vi "Open CANCoders.vi"(8 "error in":errorcluster, 11 "CANCoder Can IDs":T3={"LF ID"=12, "LB ID"=11, "RF ID"=10, "RB ID"=9}) -> (0 "error out":errorcluster, 3 "Swerve CANCoders":T1)   [LabVIEW 2020]
uses:
  Type Definitions/Hardware/4 Absolute Encoder Sets/(CANcoder) 4 Absolute Encoder Set.ctl
  <vilib>/Rock Robotics/WPI/ThirdParty/Phoenix-LabVIEW/CANCoder/Controls/CTRE_Phoenix_CANcoder_DeviceRef.ctl
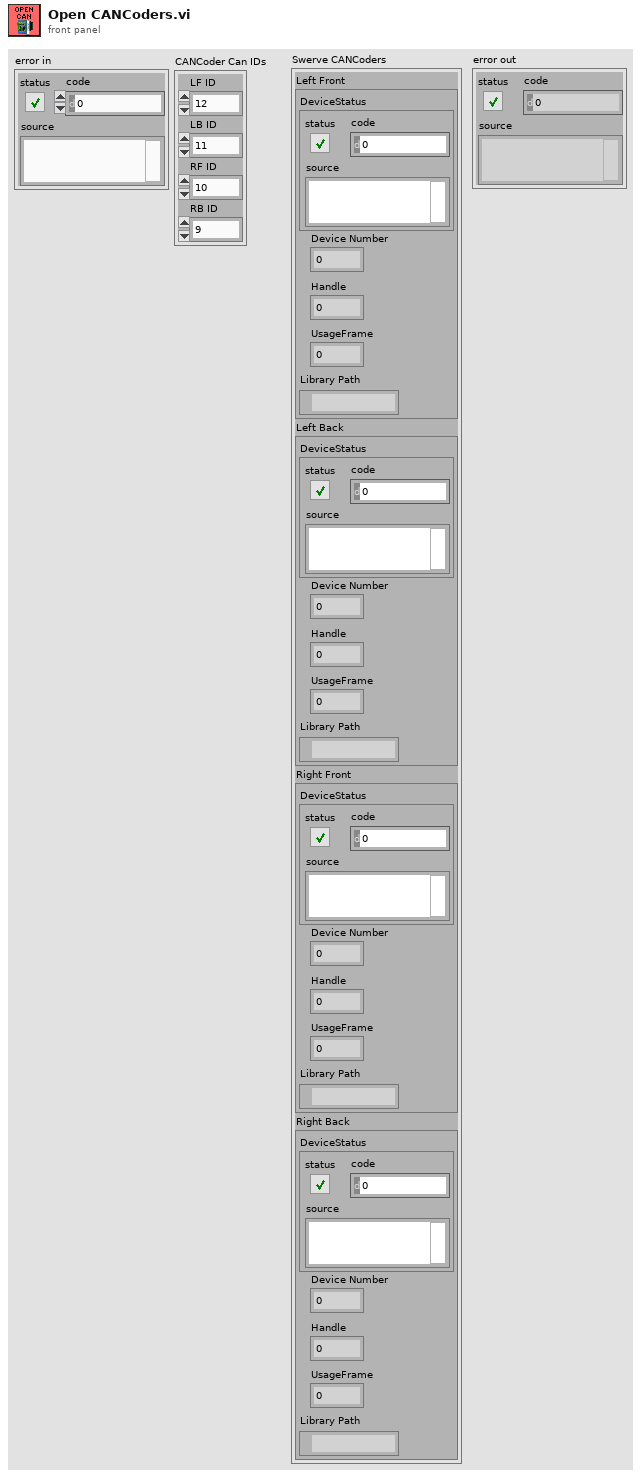
[diagram p1: front panel]
types:
  T1 = typedef "(CANcoder) 4 Absolute Encoder Set.ctl" = cluster{"Left Front":T2, "Left Back":T2, "Right Front":T2, "Right Back":T2}
  T2 = typedef "CTRE_Phoenix_CANcoder_DeviceRef.ctl" = cluster{"DeviceStatus":errorcluster, "Device Number":u8, "Handle":u64, "UsageFrame":u32, "Library Path":path}
  T3 = cluster{"LF ID":u8, "LB ID":u8, "RF ID":u8, "RB ID":u8}
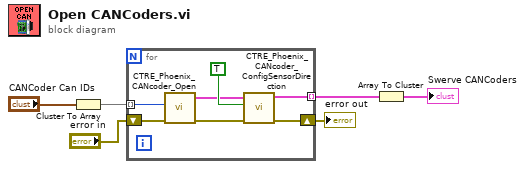
[diagram p0: block diagram]
diagram:
  n1 = Cluster To Array(cluster="CANCoder Can IDs") -> (array=w5:u8[])
  n2 = for {
    tunnel: w5 -> [w13] mode=indexing
    shift-right: [w8] -> w3
    shift-left: "error in" -> [w12]
    tunnel: [w9] -> w2 mode=indexing
    n3 = call <vilib>:"CTRE_Phoenix_CANcoder_Open.vi"("error in"=w12, "Device Number"=w13) -> ("error out"=w7:errorcluster, "CTRE_CANcoder_DeviceRef"=w10:T2)  [unwired: 8 in]
    n4 = call <vilib>:"CTRE_Phoenix_CANcoder_ConfigSensorDirection.vi"("error in"=w7, "Sensor Direction"=TRUE, "CTRE_CANcoder_DeviceRef"=w10) -> ("error out"=w8:errorcluster, "CTRE_CANcoder_DeviceRef"=w9:T2)  [unwired: 7 in]
  }
  "error out" <- w3
  n5 = Array To Cluster(array=w2) -> (cluster=→"Swerve CANCoders":cluster{"[0]":T2, "[1]":T2, "[2]":T2, "[3]":T2})
